vi "BLDC Drive State.vi"(3 "BLDC State":T1(ring), 4 "CW":bool) -> (0 "C":enum16{"H", "L", "Z"}(ring), 1 "B":enum16{"H", "L", "Z"}(ring), 2 "A":enum16{"H", "L", "Z"}(ring))   [LabVIEW 2019]
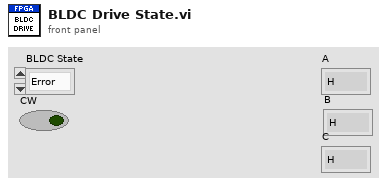
[diagram p1: front panel]
types:
  T1 = enum16{"Error", "Step 1", "Step 2", "Step 3", "Step 4", "Step 5", "Step 6"}
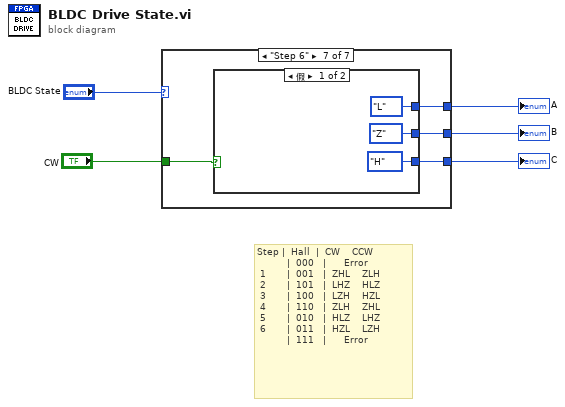
[diagram p0: block diagram]
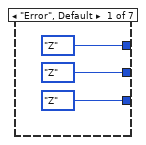
[diagram p2: hidden frame]
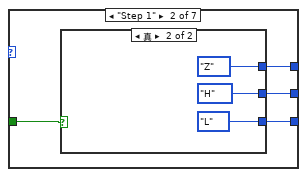
[diagram p3: hidden frame]
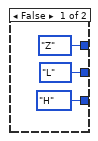
[diagram p4: hidden frame]
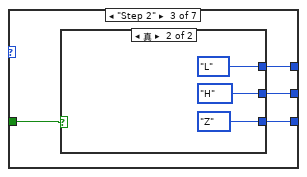
[diagram p5: hidden frame]
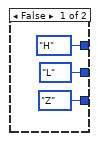
[diagram p6: hidden frame]
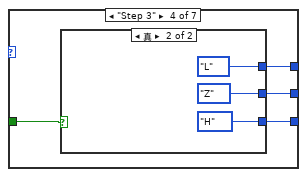
[diagram p7: hidden frame]
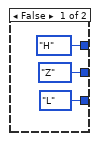
[diagram p8: hidden frame]
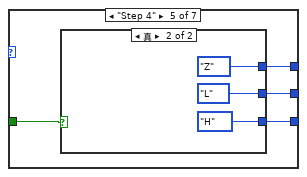
[diagram p9: hidden frame]
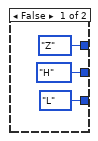
[diagram p10: hidden frame]
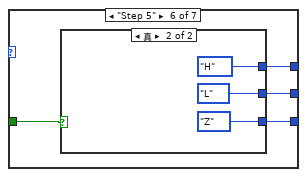
[diagram p11: hidden frame]
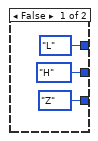
[diagram p12: hidden frame]
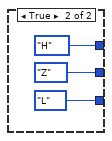
[diagram p13: hidden frame]
diagram:
  # "Step |  Hall  |  CW    CCW\n          |  000   |      Error\n 1       |  001   |  ZHL    ZLH\n 2       |  101   |  LHZ    HLZ\n 3       |  100   |  LZH    HZL\n 4       |  110   |  ZLH    ZHL\n 5       |  010   |  HLZ    LHZ\n 6       |  011   |  HZL    LZH\n          |  111   |      Error"
  n1 = case shown="\"Step 6\"" "BLDC State" {
    tunnel: [enum16{"H", "L", "Z"}."Z" w12 w22 w32 w42 w52 w62] -> w4
    tunnel: [enum16{"H", "L", "Z"}."Z" w11 w21 w31 w41 w51 w61] -> w3
    tunnel: [enum16{"H", "L", "Z"}."Z" w10 w20 w30 w40 w50 w60] -> w2
    tunnel: "CW" -> [_ w9 w19 w29 w39 w49 w59]
    frame "Error", Default {
    }
    frame "Step 1" {
      n2 = case shown="真" w9 {
        tunnel: [enum16{"H", "L", "Z"}."Z" enum16{"H", "L", "Z"}."Z"] -> w12
        tunnel: [enum16{"H", "L", "Z"}."L" enum16{"H", "L", "Z"}."H"] -> w11
        tunnel: [enum16{"H", "L", "Z"}."H" enum16{"H", "L", "Z"}."L"] -> w10
        frame False {
        }
        frame True {
        }
      }
    }
    frame "Step 2" {
      n3 = case shown="真" w19 {
        tunnel: [enum16{"H", "L", "Z"}."H" enum16{"H", "L", "Z"}."L"] -> w22
        tunnel: [enum16{"H", "L", "Z"}."L" enum16{"H", "L", "Z"}."H"] -> w21
        tunnel: [enum16{"H", "L", "Z"}."Z" enum16{"H", "L", "Z"}."Z"] -> w20
        frame False {
        }
        frame True {
        }
      }
    }
    frame "Step 3" {
      n4 = case shown="真" w29 {
        tunnel: [enum16{"H", "L", "Z"}."H" enum16{"H", "L", "Z"}."L"] -> w32
        tunnel: [enum16{"H", "L", "Z"}."Z" enum16{"H", "L", "Z"}."Z"] -> w31
        tunnel: [enum16{"H", "L", "Z"}."L" enum16{"H", "L", "Z"}."H"] -> w30
        frame False {
        }
        frame True {
        }
      }
    }
    frame "Step 4" {
      n5 = case shown="真" w39 {
        tunnel: [enum16{"H", "L", "Z"}."Z" enum16{"H", "L", "Z"}."Z"] -> w42
        tunnel: [enum16{"H", "L", "Z"}."H" enum16{"H", "L", "Z"}."L"] -> w41
        tunnel: [enum16{"H", "L", "Z"}."L" enum16{"H", "L", "Z"}."H"] -> w40
        frame False {
        }
        frame True {
        }
      }
    }
    frame "Step 5" {
      n6 = case shown="真" w49 {
        tunnel: [enum16{"H", "L", "Z"}."L" enum16{"H", "L", "Z"}."H"] -> w52
        tunnel: [enum16{"H", "L", "Z"}."H" enum16{"H", "L", "Z"}."L"] -> w51
        tunnel: [enum16{"H", "L", "Z"}."Z" enum16{"H", "L", "Z"}."Z"] -> w50
        frame False {
        }
        frame True {
        }
      }
    }
    frame "Step 6" {
      n7 = case shown="假" w59 {
        tunnel: [enum16{"H", "L", "Z"}."L" enum16{"H", "L", "Z"}."H"] -> w62
        tunnel: [enum16{"H", "L", "Z"}."Z" enum16{"H", "L", "Z"}."Z"] -> w61
        tunnel: [enum16{"H", "L", "Z"}."H" enum16{"H", "L", "Z"}."L"] -> w60
        frame False {
        }
        frame True {
        }
      }
    }
  }
  "A" <- w4
  "B" <- w3
  "C" <- w2
